vi "SampleMaster.vi"() -> ()   [LabVIEW 2012]
doc: "A sample master that can be run on the computer or RIO"
uses:
  <userlib>/ROSforLV/ROS/Code/SubVIs/_ROSControl.ctl
  <userlib>/ROSforLV/ROS/Code/SubVIs/_ROSDirection.ctl
panel:
  in  "Show Web":bool
  in  "Show Node":bool
  out "Answer":string
  in  "LED":bool
  out "LED reply":string
  out "time":string
  out "Status":string
  in  "stop":bool
  # "Instructions:\n1. Run the VI\n2. Verify that you see the correct time.\n3. Press the LED button. You should see the LED reply change.\nIf you are targetting a myRIO, the LED should change as well.\n4. Debug by clicking Show Node and Show Webpage.\n5. See what is being sent back and forth by clicking Show Node and Show Webpage."
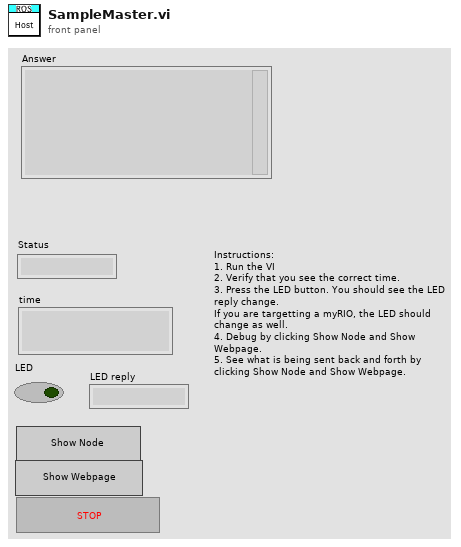
[diagram p1: front panel]
types:
  T1 = typedef "_ROSControl.ctl" = cluster{"topic port":u16, "Node":string, "topic":string, "type":string, "node port":u16, "error ":errorcluster, "Direction":T2, "Update (ms)":u16, "queue size":u16}
  T2 = typedef "_ROSDirection.ctl" = enum16{"Node", "Publisher", "Subscriber", "Service Client"}
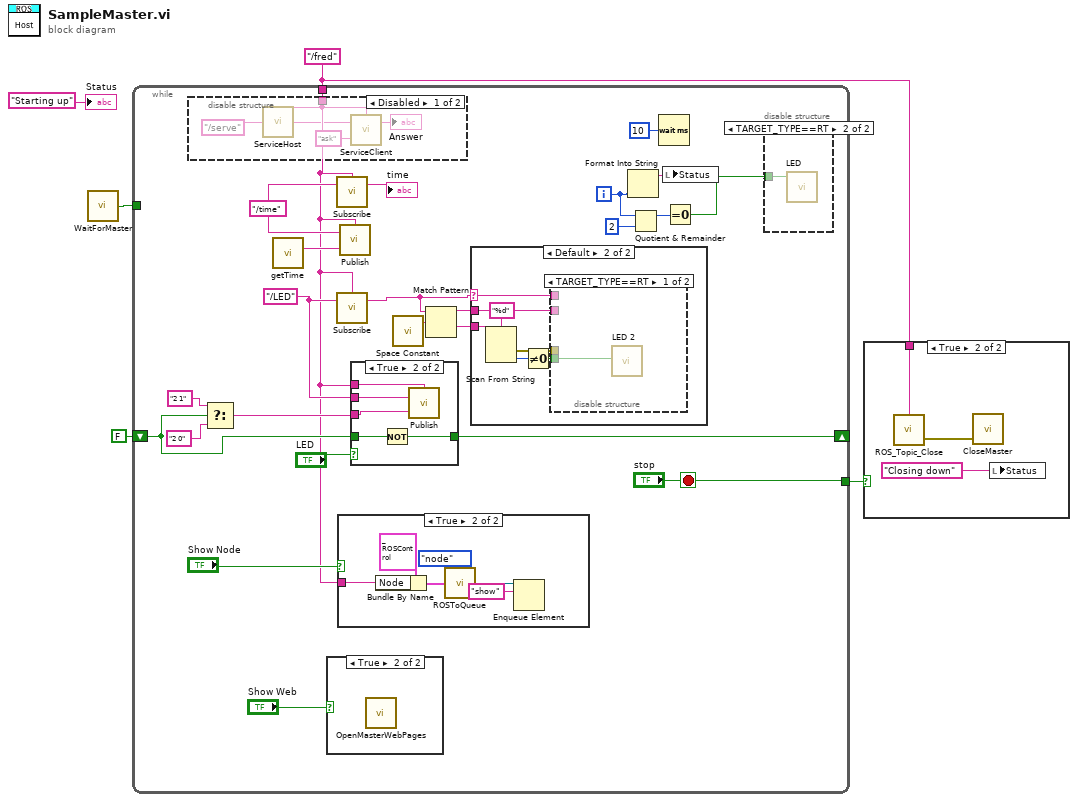
[diagram p0: block diagram]
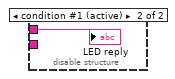
[diagram p9: hidden frame]
diagram:
  w2 = "/fred" ("Topic")
  n1 = call <userlib>:"WaitForMaster.vi"() -> ("Master There?"=w1:bool)  [unwired: 1 in]
  n2 = while {
    tunnel: ["stop"] -> w3
    tunnel: w2 -> [w11]
    shift-right: [w22] -> _
    shift-left: FALSE -> [w21]
    tunnel: w1 -> [_]
    i -> [w9]
    stop <- "stop" stop-if-true
    w15 = "/LED" ("Topic")
    w12 = "/time" ("Topic")
    n3 = disable-structure shown="Disabled" {
      disable-tunnel: w11 -> [w44 _]
      frame Disabled {
        w43 = "/serve" ("Topic")
        n4 = call <userlib>:"ServiceHost.vi"("Topic"=w43, "node"=w44) -> ()  [unwired: 1 in, 2 out]
        n5 = call <userlib>:"ServiceClient.vi"("Msg in"="ask", "Topic"=w43, "node"=w44) -> ("Reply"=→"Answer":string)  [unwired: 1 out]
      }
      frame Enabled {
      }
    }
    n6 = Select(t="2 1" ("Status"), s=w21, f="2 0" ("Status")) -> (s? t:f=w23:string)
    n7 = call <userlib>:"getTime.vi"() -> ("Current Time"=w13:string)  [unwired: 1 in]
    n8 = case shown="True" "Show Web" {
      frame False {
      }
      frame True {
        n9 = call <userlib>:"OpenMasterWebPages.vi"() -> ()  [unwired: 4 in]
      }
    }
    n10 = call <userlib>:"Subscribe.vi"("Topic"=w12, "node"=w11) -> ("Reply"=→"time":string)  [unwired: 1 in, 1 out]
    n11 = call <userlib>:"Subscribe.vi"("Topic"=w15, "node"=w11) -> ("Reply"=w14:string)  [unwired: 1 in, 1 out]
    n12 = case shown="True" "Show Node" {
      tunnel: w11 -> [_ w41]
      frame False {
      }
      frame True {
        n13 = Bundle By Name(cluster=T1 {"topic port"=0, "Node"="/fred", "topic"="/robot/head/command_head_nod", "type"="std_msgs/Bool", "node port"=59377, "error "={"status"=FALSE, "code"=0, "source"=""}, "Direction"=enum."Publisher", "Update (ms)"=1, "queue size"=1} ("ROS"), "Node"=w41) -> (w40:T1)
        n14 = call <userlib>:"ROSToQueue.vi"("ROS"=w40, "Name"=enum16{"topic", "node"}."node") -> ("queue"=w38:refnum<queue>)  [unwired: 2 in, 1 out]
        n15 = Enqueue Element(queue=w38, element="show") -> ()  [unwired: 2 in, 3 out]
      }
    }
    n16 = call <userlib>:"Publish.vi"("String"=w13, "Topic"=w12, "node"=w11) -> ()  [unwired: 1 in, 1 out]
    n17 = case shown="True" "LED" {
      tunnel: w11 -> [_ w33]
      tunnel: w15 -> [_ w34]
      tunnel: w23 -> [_ w32]
      tunnel: [w31 w35] -> w22
      tunnel: w21 -> [w31 w36]
      frame False {
      }
      frame True {
        n18 = Not(x=w36) -> (.not. x?=w35:bool)
        n19 = call <userlib>:"Publish.vi"("String"=w32, "Topic"=w34, "node"=w33) -> ()  [unwired: 1 in, 1 out]
      }
    }
    n20 = call <vilib>:"Space Constant.vi"() -> ("String"=w18:string)
    n21 = Match Pattern(string=w14, regular expression=w18) -> (before substring=w27:string, after substring=w26:string)  [unwired: 1 in, 2 out]
    n22 = case shown="Default" w14 {
      selector: w14 -> [_ w47]
      tunnel: w27 -> [_ w53]
      tunnel: w26 -> [_ w52]
      frame "" {
      }
      frame Default {
        n23 = Scan From String(format string="%d", input string=w52) -> (error out=w48:errorcluster, output 1=w50:i32)  [unwired: 3 in, 2 out]
        n24 = Not Equal To 0?(x=w50) -> (x != 0?=w49:bool)
        n25 = disable-structure shown="TARGET_TYPE==RT" {
          disable-tunnel: w53 -> [_ _]
          disable-tunnel: w49 -> [w54 _]
          disable-tunnel: w48 -> [_ _]
          disable-tunnel: w47 -> [_ w55]
          frame condition #0 {
            n26 = call "LED 2"("LED0"=w54) -> ()  [unwired: 26 in, 1 out]
          }
          frame condition #1 (active) {
            "LED reply" <- w55
          }
        }
      }
    }
    n27 = Format Into String(w9) -> (resulting string=w28:string)  [unwired: 3 in, 1 out]
    n28 = Quotient & Remainder(x=w9, y=2) -> (x-y*floor(x/y)=w7:i32)  [unwired: 1 out]
    n29 = Wait (ms)(milliseconds to wait=u32 10) -> ()  [unwired: 1 out]
    n30 = local write "Status"(w28) -> ()
    n31 = Equal To 0?(x=w7) -> (x = 0?=w6:bool)
    n32 = disable-structure shown="TARGET_TYPE==RT" {
      disable-tunnel: w6 -> [_ w30]
      frame condition #0 (active) {
      }
      frame condition #1 {
        n33 = call "LED"("LED2"=w30) -> ()  [unwired: 26 in, 1 out]
      }
    }
  }
  n34 = case shown="True" w3 {
    tunnel: w2 -> [_ w57]
    frame False {
    }
    frame True {
      n35 = call <userlib>:"ROS_Topic_Close.vi"("node"=w57) -> ("error out"=w56:errorcluster)  [unwired: 3 in]
      n36 = call <userlib>:"CloseMaster.vi"("error in (no error)"=w56) -> ()  [unwired: 2 in, 1 out]
      n37 = local write "Status"("Closing down" ("Status")) -> ()
    }
  }
  "Status" <- "Starting up" ("Status")
